vi "9237_Initialize.vi"(8 "error in (no error)":errorcluster, 9 "Slot Settings":T1, 11 "9237 in":refnum<class "9237.lvclass">) -> (0 "error out":errorcluster, 3 "9237 out":refnum<class "9237.lvclass">)   [LabVIEW 2017, in "Modules.lvlib" / "9237.lvclass"]
uses:
  9237.lvclass
  RSI Module/Slot Settings.ctl
  C:/Users/dbuck/Documents/GitHub/Scan-Engine-Custom-Device-Classes/Source/RSI Module/RSI Module.lvclass
  RSI Module/Channels.ctl
  RSI Module/Channel Type.ctl
  RSI Module/Module Models.ctl
  _nicrio_cRIO-923x_ExcitationVoltageRing.ctl
  AI Settings.ctl
  Data rate.ctl
  9237.lvclass/9237.ctl
  RSI Module/RSI Module.lvclass
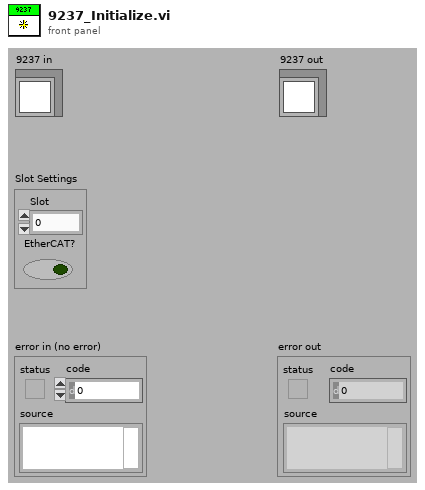
[diagram p1: front panel]
types:
  T1 = typedef "Modules.lvlib/RSI Module.lvclass/Slot Settings.ctl" = cluster{"Slot":u32, "EtherCAT?":bool}
  T2 = typedef "Modules.lvlib/9237.lvclass/AI Settings.ctl" = cluster{"AI0 Bridge":bool, "AI0 Shunt":bool, "AI1 Bridge":bool, "AI1 Shunt":bool, "AI2 Bridge":bool, "AI2 Shunt":bool, "AI3 Bridge":bool, "AI3 Shunt":bool}
  T3 = typedef "Modules.lvlib/RSI Module.lvclass/Module Models.ctl" = enum16{"Empty", "NI 9201", "NI 9203", "NI 9205", "NI 9206", "NI 9207", "NI 9208", "NI 9211", "NI 9212", "NI 9213", "NI 9214", "NI 9215", "NI 9217", "NI 9219", "NI 9220", "NI 9221", "NI 9222", "NI 9223", "NI 9225", "NI 9227", "NI 9229", "NI 9233", "NI 9234", "NI 9235", "NI 9236", "NI 9237", "NI 9239", "NI 9242", "NI 9244", "NI 9263", "NI 9264", "NI 9265", "NI 9269", "NI 9375", "NI 9401", "NI 9402", "NI 9403", "NI 9411", "NI 9421", "NI 9422", "NI 9423", "NI 9425", "NI 9426", "NI 9435", "NI 9437", "NI 9472", "NI 9474", "NI 9475", "NI 9476", "NI 9477", "NI 9478", "NI 9481", "NI 9482", "NI 9485"}
  T4 = typedef "Modules.lvlib/RSI Module.lvclass/Channels.ctl" = cluster{"# Input Channels":i32, "# Output Channels":i32, "Channel Type":T5, "Units":string}
  T5 = typedef "Modules.lvlib/RSI Module.lvclass/Channel Type.ctl" = enum16{"Analog", "Digital"}
  T6 = typedef "Modules.lvlib/9237.lvclass/Data rate.ctl" = u32
  T7 = typedef "Modules.lvlib/9237.lvclass/_nicrio_cRIO-923x_ExcitationVoltageRing.ctl" = u8
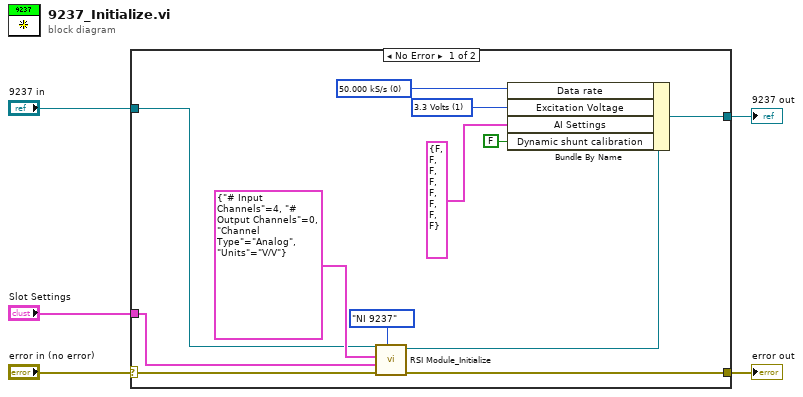
[diagram p0: block diagram]
diagram:
  n1 = case shown="No Error" "error in (no error)" {
    selector: "error in (no error)" -> [w14 w19]
    tunnel: [w13 w19] -> w4
    tunnel: [w11 w18] -> w2
    tunnel: "9237 in" -> [w16 w18]
    tunnel: "Slot Settings" -> [w15 _]
    frame No Error {
      w6 = T6 0 items=["50.000 kS/s", "25.000 kS/s", "16.667 kS/s", "12.500 kS/s", "10.000 kS/s", "8.333 kS/s", "7.143 kS/s", "6.250 kS/s", "5.556 kS/s", "5.000 kS/s", "4.545 kS/s", "4.167 kS/s", "3.846 kS/s", "3.571 kS/s", "3.333 kS/s", "3.125 kS/s", "2.941 kS/s", "2.778 kS/s", "2.632 kS/s", "2.500 kS/s", "2.381 kS/s", "2.273 kS/s", "2.174 kS/s", "2.083 kS/s", "2.000 kS/s", "1.923 kS/s", "1.852 kS/s", "1.786 kS/s", "1.724 kS/s", "1.667 kS/s", "1.613 kS/s"] ("Data rate")
      w9 = T7 1 items=["2.5 Volts", "3.3 Volts", "5.0 Volts", "10.0 Volts", "External Excitation"] ("Excitation Voltage")
      n2 = call "RSI Module_Initialize.vi"("Module Model"=Module_Models."NI 9237", "error in (no error)"=w14, "Slot Settings"=w15, "Channels"=T4 {"# Input Channels"=4, "# Output Channels"=0, "Channel Type"=enum."Analog", "Units"="V/V"}, "RSI Module in"=w16) -> ("error out"=w13:errorcluster, "RSI Module out"=w12:refnum<class "9237.lvclass">)  [unwired: 5 in]
      n3 = Bundle By Name(cluster=w12, "Data rate"=w6, "Excitation Voltage"=w9, "AI Settings"=T2 {"AI0 Bridge"=FALSE, "AI0 Shunt"=FALSE, "AI1 Bridge"=FALSE, "AI1 Shunt"=FALSE, "AI2 Bridge"=FALSE, "AI2 Shunt"=FALSE, "AI3 Bridge"=FALSE, "AI3 Shunt"=FALSE}, "Dynamic shunt calibration"=FALSE) -> (w11:refnum<class "9237.lvclass">)
    }
    frame Error {
    }
  }
  "error out" <- w4
  "9237 out" <- w2
